vi "BRig_RT_comm_webdav_upload_all__genericCheckAll.vi"(0 "input_hSession":T1, 1 "input_arrFilenames":string[](array[string]), 2 "input_n":i32, 5 "input_error":errorcluster, 7 "input_arrUploaded":bool[](array[boolean]), 9 "input_arrSentTarget":bool[](array[boolean]), 11 "input_arrSentTargetSpare":bool[](array[boolean]), 12 "input_fileName_prefix":string, 13 "input_Target(F)_or_Spare(T)":bool) -> (4 "output_hSession":T1, 6 "output_error":errorcluster, 8 "output_arrUploaded":bool[](array[boolean]), 10 "output_arrSentTarget":bool[](array[boolean]), 15 "output_arrSentTargetSpare":bool[](array[boolean]))   [LabVIEW 2014]
uses:
  <vilib>/WebDAVClient/Advanced/SessionHandle.ctl
  <vilib>/WebDAVClient/NI_WebDAV.lvlib
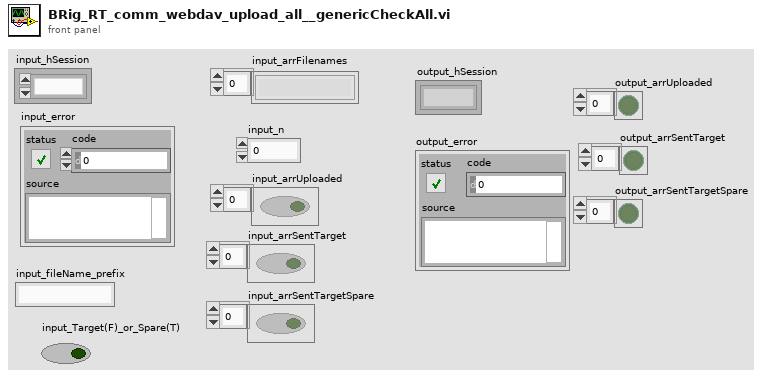
[diagram p1: front panel]
types:
  T1 = typedef "NI_WebDAV.lvlib/SessionHandle.ctl" = refnum<k1>
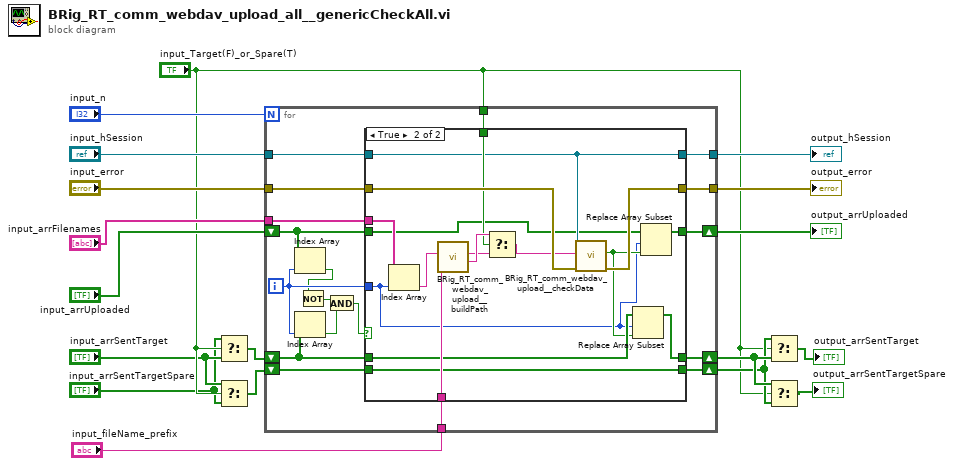
[diagram p0: block diagram]
diagram:
  n1 = Select(t="input_arrSentTargetSpare", s="input_Target(F)_or_Spare(T)", f="input_arrSentTarget") -> (s? t:f=w2:bool[])
  n2 = Select(t="input_arrSentTarget", s="input_Target(F)_or_Spare(T)", f="input_arrSentTargetSpare") -> (s? t:f=w1:bool[])
  n3 = for {
    N: "input_n" -> [_]
    tunnel: "input_arrFilenames" -> [w36]
    shift-right: [w29] -> w10
    shift-left: "input_arrUploaded" -> [w24]
    tunnel: "input_fileName_prefix" -> [w35]
    tunnel: "input_hSession" -> [w33]
    tunnel: [w30] -> w12
    tunnel: "input_error" -> [w34]
    shift-right: [w27] -> w9
    shift-left: w2 -> [w28]
    shift-right: [w25] -> w8
    shift-left: w1 -> [w26]
    tunnel: [w32] -> w11
    tunnel: "input_Target(F)_or_Spare(T)" -> [w31]
    i -> [w23]
    n4 = Index Array(array=w24, index=w23) -> (element=w22:bool)
    n5 = Index Array(array=w28, index=w23) -> (element=w20:bool)
    n6 = Not(x=w22) -> (.not. x?=w21:bool)
    n7 = And(x=w21, y=w20) -> (x .and. y?=w19:bool)
    n8 = case shown="True" w19 {
      tunnel: w36 -> [_ w58]
      tunnel: w35 -> [_ w57]
      tunnel: w34 -> [w40 w55]
      tunnel: w33 -> [w41 w49]
      tunnel: [w40 w54] -> w32
      tunnel: w31 -> [_ w50]
      tunnel: w23 -> [_ w42]
      tunnel: [w41 w49] -> w30
      tunnel: [w39 w44] -> w29
      tunnel: w24 -> [w39 w45]
      tunnel: w28 -> [w38 w48]
      tunnel: [w38 w47] -> w27
      tunnel: w26 -> [w37 w46]
      tunnel: [w37 w46] -> w25
      frame False {
      }
      frame True {
        n9 = Index Array(array=w58, index=w42) -> (element=w56:string)
        n10 = call "BRig_RT_comm_webdav_upload__buildPath.vi"("input_fileName_prefix"=w57, "input_fileName"=w56) -> ("output_targetPath_spare"=w53:string, "output_targetPath"=w52:string)  [unwired: 7 in, 1 out]
        n11 = Select(t=w53, s=w50, f=w52) -> (s? t:f=w51:string)
        n12 = call "BRig_RT_comm_webdav_upload__checkData.vi"("input_error"=w55, "input_targetPath"=w51, "input_hSession"=w49) -> ("error out"=w54:errorcluster, "output_checkData"=w43:bool)  [unwired: 6 in, 1 out]
        n13 = Replace Array Subset(array=w48, new element=w43, index=w42) -> (w47:bool[])
        n14 = Replace Array Subset(array=w45, new element=w43, index=w42) -> (w44:bool[])
      }
    }
  }
  "output_hSession" <- w12
  "output_error" <- w11
  "output_arrUploaded" <- w10
  n15 = Select(t=w8, s="input_Target(F)_or_Spare(T)", f=w9) -> (s? t:f=→"output_arrSentTarget":bool[])
  n16 = Select(t=w9, s="input_Target(F)_or_Spare(T)", f=w8) -> (s? t:f=→"output_arrSentTargetSpare":bool[])
